vi "DaqReadFFT1.vi"(6 "restart averaging (F)":bool, 8 "error in":errorcluster caption="错误输入", 9 "WFGraph引用句柄FFT":refnum<vi>, 10 "WFGraph引用句柄Order":refnum<vi>, 11 "任务输入":refnum<k21>) -> (0 "error out":errorcluster, 1 "spectrum info":T1[](array[typedef]) {"x-axis units" items=["Time (s)"=0, "Frequency-CB (Hz)"=1, "Frequency-CPB (Hz)"=1248, "Frequency-Arbitrary (Hz)"=2357, "Quefrency (s)"=2, "Revolutions (rev)"=3, "Order"=4, "Speed (RPM)"=11, "Speed (rad/s)"=21, "Index"=65535]; "weighting filter" items=["Linear", "A-weighting", "B-weighting", "C-weighting", "ITU-R 468-4", "Dolby", "CCITT", "C-message", "Wb", "Wc", "Wd", "We", "Wf", "Wh", "Wj", "Wk", "Wm", "AES17 20 kHz lowpass", "AES17 40 kHz lowpass", "AES17 20 kHz highpass", "AES17 40 kHz highpass"]; "dB reference [EU]" format="%.2f"; "engineering units" items=["custom..."=0, "V"=1, "A"=21, "C"=30, "pC"=31, "s"=32, "-"=29, "Pa"=2, "N"=20, "g"=3, "m/s^2"=4, "m/s"=5, "m"=6, "mm/s"=12, "mm"=13, "micron/s"=14, "micron"=15, "in/s^2"=7, "in/s"=8, "in"=9, "mil/s"=10, "mil"=11, "rad/s^2"=16, "rad/s"=17, "rad"=18, "deg/s^2"=26, "deg/s"=27, "deg"=28, "RPM"=22, "cycle/s^2"=23, "Hz"=24, "cycle"=25, "strain"=19]; "spectral info"."window" items=["None "=0, "Hanning"=1, "Hamming"=2, "Blackman-Harris"=3, "Exact Blackman"=4, "Blackman"=5, "Flat Top"=6, "4 Term B-Harris "=7, "7 Term B-Harris"=8, "Low Sidelobe"=9, "Force - Exponential"=10, "Gaussian"=62]}, 2 "done":bool, 3 "task out 2":refnum<k21> caption="任务输出")   [LabVIEW 2020]
uses:
  <vilib>/_NISVFA/_Shared subVIs/Controls/svc_Channel Info.ctl
  <vilib>/_NISVFA/_Shared subVIs/Controls/svc_Engineering Units Text Ring.ctl
  <vilib>/_NISVFA/_Shared subVIs/Controls/svc_Weighting Filter Text Ring.ctl
  <vilib>/_NISVFA/_Shared subVIs/Controls/svc_Window.ctl
  <vilib>/_NISVFA/_Shared subVIs/Controls/svc_Spectrum Info.ctl
  <vilib>/_NISVFA/_Shared subVIs/Controls/svc_X-Axis Units.ctl
  <vilib>/_NISVFA/_Shared subVIs/Controls/svc_Spectrum Type.ctl
  <vilib>/_NISVFA/_Shared subVIs/Controls/svc_Complimentary Spectrum Units.ctl
  <vilib>/DAQmx/read.llb/DAQmx Read (Analog 1D Wfm NChan NSamp).vi
  <vilib>/addons/Sound and Vibration/svt_Calibration/SVL Scale Voltage to EU (N Ch - 1 Info).vi
  <vilib>/addons/Sound and Vibration/svt_Calibration/SVL Scale Voltage to EU (1 Ch).vi
  <vilib>/_NISVFA/_Shared subVIs/Common/svc_Set SV Channel Info.vi
  <vilib>/_NISVFA/_Shared subVIs/Common/svc_Set SV Channel Info (variant).vi
  <vilib>/_NISVFA/_Shared subVIs/Common/SVL Set dB Reference (variant).vi
  <vilib>/DAQmx/miscellaneous.llb/DAQmx Fill In Error Info.vi
  <vilib>/_NISVFA/_Shared subVIs/Common/svc_Engineering Units to Unit Label.vi
  <vilib>/_NISVFA/_Shared subVIs/Common/svc_Compute Scale Factor to Convert V to EU.vi
  <vilib>/_NISVFA/_Shared subVIs/Common/svc_Compute Scale Factor to Convert C to EU.vi
  <vilib>/_NISVFA/_Shared subVIs/Common/svc_Set dB ref if Pascal.vi
  <vilib>/_NISVFA/_Shared subVIs/Common/svc_Caller VI Returned in Error Source.vi
  <vilib>/_NISVFA/_Subset FFT/SVFA Power Spectrum Subset (N Ch).vi
  <vilib>/addons/Sound and Vibration/svt_Calibration/SoundVib_Calibration.lvlib
panel:
  in  "frequency range":T7={"start frequency"=0.0, "stop frequency"=20000.0} {"stop frequency" min=0.0 format="%.2f"; "start frequency" min=0.0 format="%.2f"}
  in  "averaging parameters":T8={"averaging mode"=enum."RMS averaging", "weighting mode"=enum."Linear", "number of averages"=200, "linear mode"=enum."One shot"} {"number of averages" min=1 step=1}
  out "averages completed":dbl
  in  "number of samples":i32=2000 min=128
  in  "dB On":bool=TRUE
  in  "window":T9=1 items=["None"=0, "Hanning"=1, "Hamming"=2, "Blackman-Harris"=3, "Exact Blackman"=4, "Blackman"=5, "Flat Top"=6, "4 Term B-Harris "=7, "7 Term B-Harris"=8, "Low Sidelobe"=9, "Blackman Nuttall"=11, "Triangle"=30, "Bartlett-Hanning"=31, "Bohman"=32, "Parzen"=33, "Welch"=34, "Kaiser"=60, "Dolph-Chebyshev"=61, "Gaussian"=62]
  in  "channel info":T10={"sensor sensitivity"=1000.0, "engineering units"=3, "dB reference"=2e-05, "custom label"="EU", "weighting filter"=0, "pregain"=0.0} {"pregain" format="%.2f"; "weighting filter" items=["Linear", "A-weighting", "B-weighting", "C-weighting", "ITU-R 468-4", "Dolby", "CCITT", "C-message", "Wb", "Wc", "Wd", "We", "Wf", "Wh", "Wj", "Wk", "Wm", "AES17 20 kHz lowpass", "AES17 40 kHz lowpass", "AES17 20 kHz highpass", "AES17 40 kHz highpass"]; "dB reference" format="%^.1e"; "engineering units" items=["custom..."=0, "V"=1, "A"=21, "C"=30, "pC"=31, "s"=32, "-"=29, "Pa"=2, "N"=20, "g"=3, "m/s^2"=4, "m/s"=5, "m"=6, "mm/s"=12, "mm"=13, "micron/s"=14, "micron"=15, "in/s^2"=7, "in/s"=8, "in"=9, "mil/s"=10, "mil"=11, "rad/s^2"=16, "rad/s"=17, "rad"=18, "deg/s^2"=26, "deg/s"=27, "deg"=28, "RPM"=22, "cycle/s^2"=23, "Hz"=24, "cycle"=25, "strain"=19]; "sensor sensitivity" format="%#_5f"}
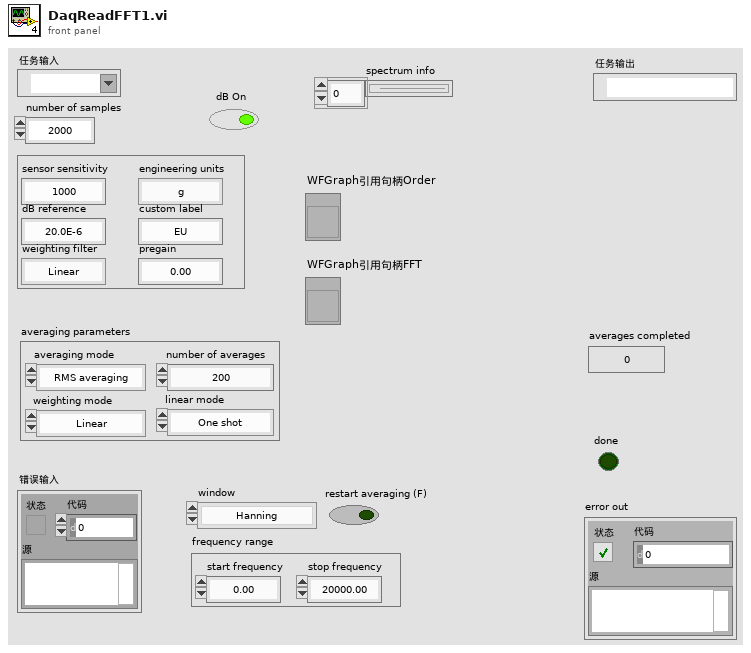
[diagram p1: front panel]
types:
  T1 = typedef "svc_Spectrum Info.ctl" = cluster{"channel name":string, "description":string, "x-axis units":T2, "spectral info":cluster{"spectrum type":T3, "linear/dB":enum16{"linear", "dB"}, "window":u16, "window size":i32, "FFT size":i32}, "engineering units":T4, "custom label":string, "dB reference [EU]":dbl, "peak units":enum16{"rms", "peak", "peak-peak"}, "weighting filter":T5, "spectral density?":bool, "unit label":string, "spectrum skewed?":bool, "complimentary spectrum units":T6}
  T2 = typedef "svc_X-Axis Units.ctl" = u16
  T3 = typedef "svc_Spectrum Type.ctl" = enum16{"FFT Spectrum [complex]", "Amplitude [Magnitude]", "Power [Magnitude^2]", "Cross Spectrum [complex]", "Frequency Response [Complex]"}
  T4 = typedef "svc_Engineering Units Text Ring.ctl" = u16
  T5 = typedef "svc_Weighting Filter Text Ring.ctl" = u16
  T6 = typedef "svc_Complimentary Spectrum Units.ctl" = enum16{"none", "radians", "degrees", "cycles", "imaginary"}
  T7 = cluster{"start frequency":dbl, "stop frequency":dbl}
  T8 = cluster{"averaging mode":enum16{"No averaging", "Vector averaging", "RMS averaging", "Peak hold"}, "weighting mode":enum16{"Linear", "Exponential"}, "number of averages":u32, "linear mode":enum16{"One shot", "Auto restart"}}
  T9 = typedef "svc_Window.ctl" = u32
  T10 = typedef "svc_Channel Info.ctl" = cluster{"sensor sensitivity":dbl, "engineering units":T4, "dB reference":dbl, "custom label":string, "weighting filter":T5, "pregain":dbl}
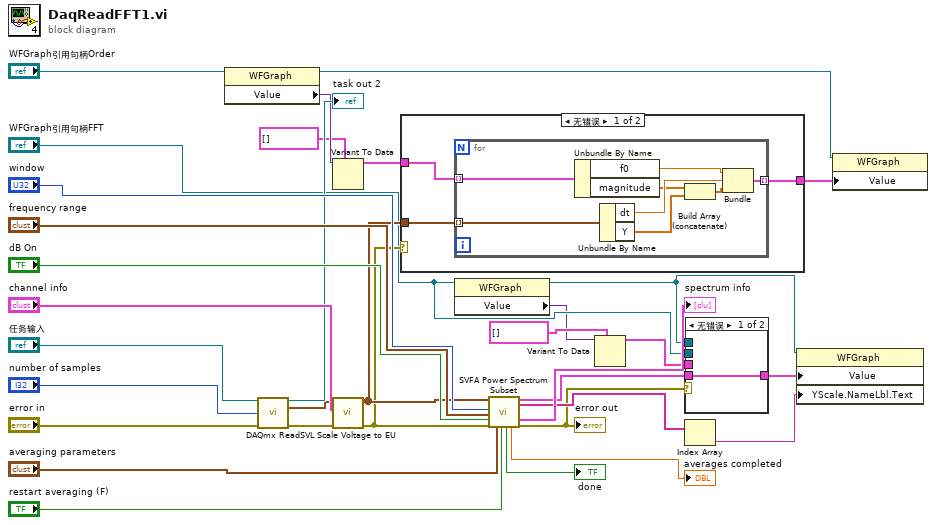
[diagram p0: block diagram]
diagram:
  n1 = property class="WFGraph"(reference="WFGraph引用句柄Order") -> (reference out=w19:refnum<vi>, "Value"=w12:variant)  [unwired: 1 in, 1 out]
  n2 = call-poly <vilib>:"DAQmx Read.vi"("task/channels in"="任务输入", "number of samples per channel"="number of samples", "error in"="error in") -> ("task out"=→"task out 2":refnum<k21>, "data"=w23:waveform(dbl)[], "error out"=w26:errorcluster)  [unwired: 10 in]
  n3 = Variant To Data(type=cluster{"f0":dbl, "df":dbl, "magnitude":dbl[]}[] [] ("波形图"), Variant=w12) -> (data=w10:cluster{"f0":dbl, "df":dbl, "magnitude":dbl[]}[])  [unwired: 1 in, 1 out]
  n4 = call-poly <vilib>:"SVL Scale Voltage to EU.vi"("error in (no error)"=w26, "channel info"="channel info", "signals [V]"=w23) -> ("error out"=w9:errorcluster, "scaled signals [EU]"=w14:waveform(dbl)[])  [unwired: 6 in, 1 out]
  n5 = case shown="无错误" w9 {
    tunnel: w14 -> [w36 _]
    tunnel: [w35 w45] -> w13
    tunnel: w10 -> [w34 w45]
    frame No Error {
      n6 = for {
        tunnel: w36 -> [w44] mode=indexing
        tunnel: [w42] -> w35 mode=indexing
        tunnel: w34 -> [w41] mode=indexing
        n7 = Unbundle By Name(w41) -> ("f0"=w40:dbl, "magnitude"=w37:dbl[])
        n8 = Unbundle By Name(w44) -> ("dt"=w43:dbl, "Y"=w38:dbl[])
        n9 = Build Array (concatenate)(w37, w38) -> (w39:dbl[])
        n10 = Bundle("f0"=w40, "dt"=w43, w39) -> (w42:cluster{"f0":dbl, "dt":dbl, dbl[]})  [unwired: 1 in]
      }
    }
    frame Error {
    }
  }
  n11 = property class="WFGraph"(reference="WFGraph引用句柄FFT") -> (reference out=w7:refnum<vi>, "Value"=w3:variant)  [unwired: 1 in, 1 out]
  n12 = call-poly <vilib>:"SVFA Power Spectrum Subset.vi"("scaled signals [EU]"=w14, "window"="window", "frequency range"="frequency range", "dB On (T)"="dB On", "error in (no error)"=w9, "averaging parameters"="averaging parameters", "restart averaging (F)"="restart averaging (F)") -> ("averaging done"=→"done":bool, "averages completed"=→"averages completed":dbl, "power spectra [dB EU]"=w16:cluster{"f0":dbl, "df":dbl, "magnitude":dbl[]}[], "unit labels"=w15:string[], "spectrum info"=→"spectrum info":T1[], "error out"=w6:errorcluster)  [unwired: 7 in]
  "error out" <- w6
  n13 = Variant To Data(type=cluster{"f0":dbl, "df":dbl, "magnitude":dbl[]}[] [] ("波形图"), Variant=w3) -> (data=w2:cluster{"f0":dbl, "df":dbl, "magnitude":dbl[]}[])  [unwired: 1 in, 1 out]
  n14 = case shown="无错误" w6 {
    tunnel: w16 -> [w46 _]
    tunnel: "WFGraph引用句柄FFT" -> [_ _]
    tunnel: w7 -> [_ _]
    tunnel: [w46 w47] -> w5
    tunnel: w2 -> [_ w47]
    frame No Error {
    }
    frame Error {
    }
  }
  n15 = Index Array(array=w15) -> (element=w1:string)  [unwired: 1 in]
  n16 = property class="WFGraph"(reference=w7, "Value"=w5, "YScale.NameLbl.Text"=w1) -> ()  [unwired: 1 in, 2 out]
  n17 = property class="WFGraph"(reference=w19, "Value"=w13) -> ()  [unwired: 1 in, 2 out]
